vi "Simulated HW Control Panel.vi"() -> ()   [LabVIEW 2017, in "Simulated HW.lvclass"]
uses:
  Simulated HW.lvclass
panel:
  in  "Cylinder 2 State":bool
  in  "Cylinder 1 State":bool
  in  "Bottom Outer Heater Temp":dbl
  in  "Bottom Inner Heater Temp":dbl
  in  "Top Outer Heater Temp":dbl
  in  "Top Inner Heater Temp":dbl
  in  "Sheet Temp":dbl
  in  "Motor Direction":bool
  in  "Motor Power":bool
  in  "Unloading Position":bool
  in  "Heating Position":bool
  in  "Loading Position":bool
  # "Limit Switches"
  # "Motor"
  # "IR Temperature Sensors"
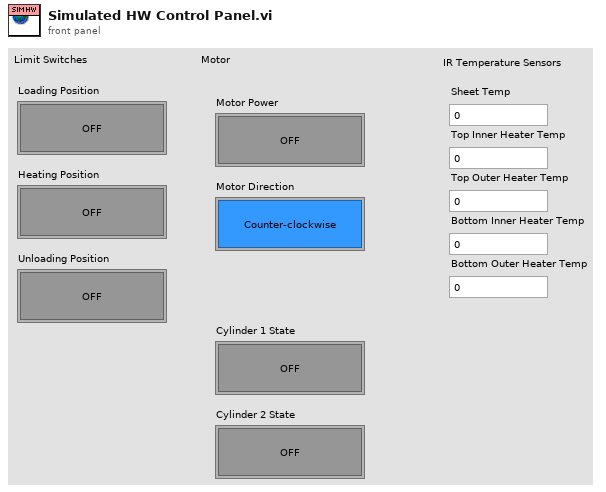
[diagram p1: front panel]
diagram:
